vi "Collate Group Channels.vi"(10 "Channel Names":string[](array[string]), 11 "Historian Module in":refnum<class "Historian Module.lvclass">) -> (1 "Unknown Channels":string[](array[string]), 2 "Grouped Channels":map{string, string[]}(c390), 3 "Historian Module out":refnum<class "Historian Module.lvclass">)   [LabVIEW 2020, in "VolatusHistorian.lvlib" / "Historian Module.lvclass"]
uses:
  Historian Module.lvclass
  Historian Module.lvclass/Historian Module.ctl
  <vilib>/Utility/miscctls.llb/LVMapReplaceAction.ctl
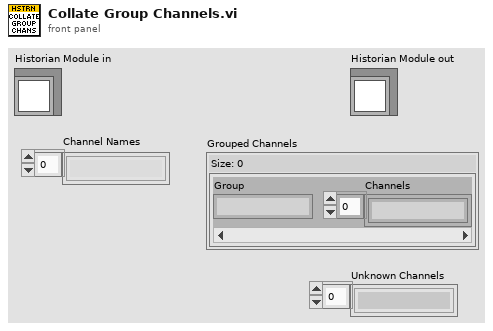
[diagram p1: front panel]
types:
  T1 = typedef "LVMapReplaceAction.ctl" = enum32{"Modify Entry only if found", "Add or Modify Entry", "Delete Entry"}
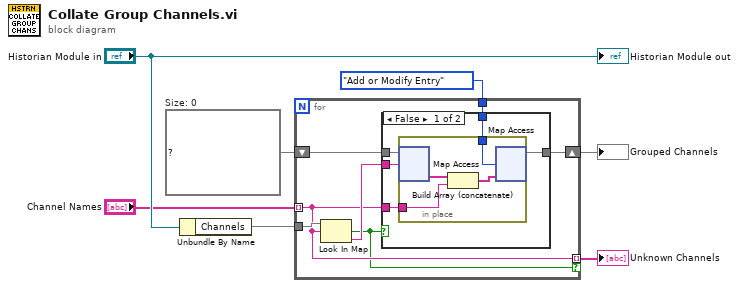
[diagram p0: block diagram]
diagram:
  w6 = map{string, string[]} {}  # Size: 0
  n1 = Unbundle By Name("Historian Module in") -> ("Channels"=w5:map{string, string})
  n2 = for {
    shift-right: [w10] -> w2
    shift-left: w6 -> [w12]
    tunnel: w5 -> [w14]
    tunnel: "Channel Names" -> [w11] mode=indexing
    tunnel: [w11] -> w1 mode=indexing if=w8
    tunnel: LVMapReplaceAction."Add or Modify Entry" ("action") -> [w9]
    n3 = Look In Map(map=w14, key=w11) -> (key not found?=w8:bool, value=w13:string)  [unwired: 1 in]
    n4 = case shown="False" w8 {
      tunnel: w13 -> [w19 _]
      tunnel: w12 -> [w18 w24]
      tunnel: w11 -> [w17 _]
      tunnel: [w16 w24] -> w10
      tunnel: w9 -> [w15 _]
      frame False {
        n5 = in-place {
          in-place-border: w17 -> [w22]
          in-place-border: w15 -> [w20]
          n6 = in-place-map #1(w18, w19) -> (w23:string[])  [unwired: 1 in, 1 out]
          n7 = Build Array (concatenate)(w23, w22) -> (w21:string[])
          n8 = in-place-map #1(w21, w20) -> (w16:map{string, string[]})  [unwired: 2 out]
        }
      }
      frame True {
      }
    }
  }
  "Grouped Channels" <- w2
  "Unknown Channels" <- w1
  "Historian Module out" <- "Historian Module in"
